vi "Status.vi"(0 "Instrument Handle In":i32, 1 "Register Type":i32(ring) items=["Event", "Condition"], 5 "error in":errorcluster) -> (8 "Dig2 Register":i32 caption="Digitizer 2 Register" format="%.0x", 9 "Dig1 Register":i32 caption="Digitzer 1 Register" format="%.0x", 10 "Calibration Register":i32 format="%.0x", 11 "Voltage Register":i32 format="%.0x", 12 "Questionable Register":i32 format="%.0x", 13 "Standard Register":i32 format="%.0x", 14 "Instrument Handle Out":i32, 15 "Status Register":i32 format="%.0x", 16 "Frequency Register":i32 format="%.0x", 17 "Test Register":i32 format="%.0x", 18 "Operation Register":i32 format="%.0x", 19 "error out":errorcluster)   [LabVIEW 8.6, in "ZTScopeM.lvlib"]
doc: "Query the event status or the present conditions of the status registers."
uses:
  ZTScopeM.lvlib
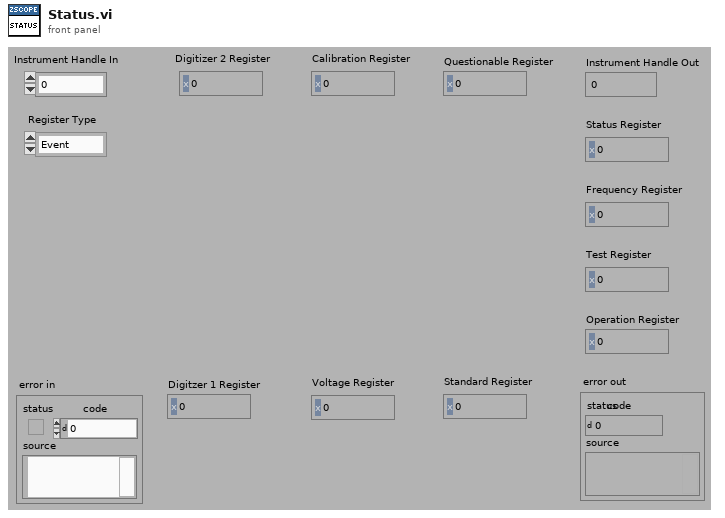
[diagram p1: front panel]
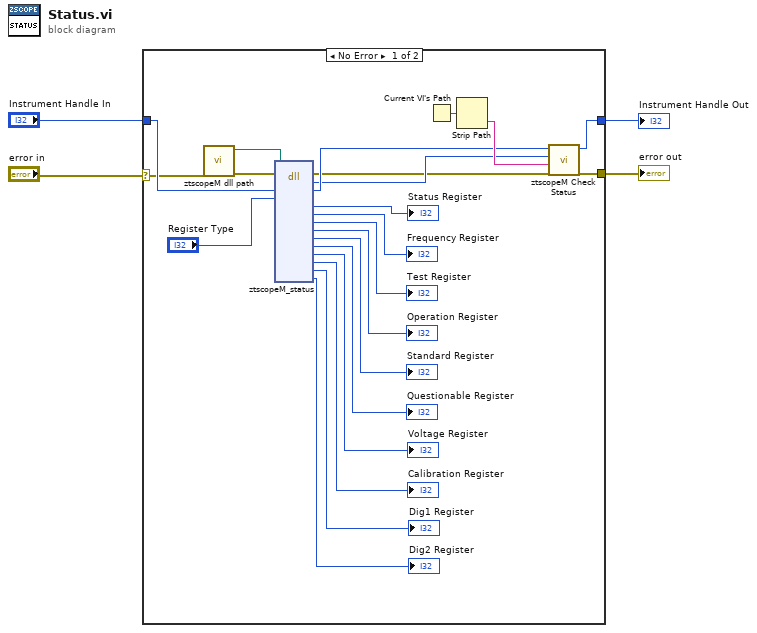
[diagram p0: block diagram]
diagram:
  n1 = case shown="No Error" "error in" {
    selector: "error in" -> [w8 w28]
    tunnel: [w11 w28] -> w1
    tunnel: "Instrument Handle In" -> [w26 w27]
    tunnel: [w12 w27] -> w3
    frame #0 {
      n2 = call "ztscopeM dll path.vi"("error in (no error)"=w8) -> ("error out"=w6:errorcluster, "<instrument>.dll path"=w7:path)  [unwired: 9 in]
      n3 = dll-call lib="C:/Program Files (x86)/National Instruments/LabVIEW 2013/instr.lib/ztscopem/ztscopeM.dll" fn="ztscopeM_status"(path in=w7, error in=w6, "instrumentHandle"=w26, "registerType"="Register Type") -> (error out=w5:errorcluster, w13:i32, "instrumentHandle"=w14:i32, "statusRegister"=→"Status Register":i32, "frequencyRegister"=→"Frequency Register":i32, "testRegister"=→"Test Register":i32, "operationRegister"=→"Operation Register":i32, "standardRegister"=→"Standard Register":i32, "questionableRegister"=→"Questionable Register":i32, "voltageRegister"=→"Voltage Register":i32, "calibrationRegister"=→"Calibration Register":i32, "dig1Register"=→"Dig1 Register":i32, "dig2Register"=→"Dig2 Register":i32)  [unwired: 12 in, 1 out]
      n4 = Current VI's Path() -> (path=w16:path)
      n5 = Strip Path(path=w16) -> (name=w15:string)  [unwired: 1 out]
      n6 = call "ztscopeM Check Status.vi"("error in"=w5, "name of VI"=w15, "status (return code)"=w13, "instrument handle in"=w14) -> ("error out"=w11:errorcluster, "instrument handle out"=w12:i32)  [unwired: 2 in]
    }
    frame #1 {
    }
  }
  "Instrument Handle Out" <- w3
  "error out" <- w1
